vi "Report Error to Process.vi"(8 "Error":errorcluster, 11 "This VI":refnum<vi>) -> ()   [LabVIEW 2014, in "Waveform-Processing-Custom-Device Engine.lvlib" / "Error Handling API.lvlib"]
uses:
  Error Handling API.lvlib
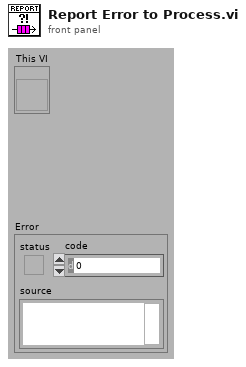
[diagram p1: front panel]
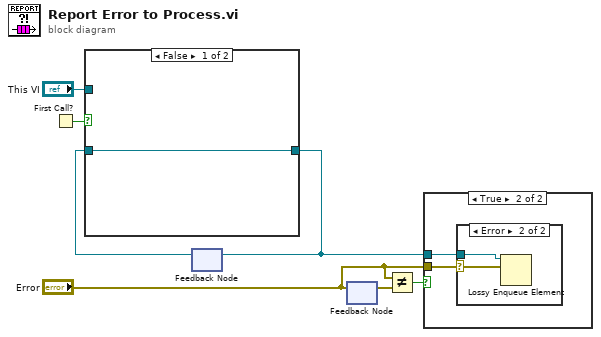
[diagram p0: block diagram]
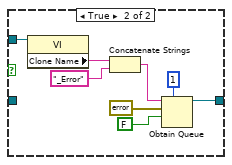
[diagram p4: hidden frame]
diagram:
  n1 = First Call?() -> (First Call?: T/F=w7:bool)
  n2 = feedback #1() -> (w5:refnum<queue>)  [unwired: 1 in]
  n3 = case shown="False" w7 {
    tunnel: "This VI" -> [_ w16]
    tunnel: [w8 w9] -> w1
    tunnel: w5 -> [w8 _]
    frame False {
    }
    frame True {
      n4 = property class="VI"(reference=w16) -> ("Clone Name"=w15:string)  [unwired: 1 in, 2 out]
      n5 = Concatenate Strings(w15, "_Error" ("string")) -> (w13:string)
      n6 = Obtain Queue(max queue size (-1, unlimited)=1, name (unnamed)=w13, element data type=errorcluster {"status"=FALSE, "code"=0, "source"=""} ("error out"), create if not found? (T)=FALSE) -> (queue out=w9:refnum<queue>)  [unwired: 1 in, 2 out]
    }
  }
  n7 = feedback-in #1(w1) -> ()
  n8 = feedback #2() -> (w3:errorcluster)  [unwired: 1 in]
  n9 = feedback-in #2("Error") -> ()
  n10 = Not Equal?(x="Error", y=w3) -> (x != y?=w4:bool)
  n11 = case shown="True" w4 {
    tunnel: w1 -> [_ w18]
    tunnel: "Error" -> [_ w17]
    frame False {
    }
    frame True {
      n12 = case shown="Error" w17 {
        selector: w17 -> [_ w19]
        tunnel: w18 -> [_ w20]
        frame No Error {
        }
        frame Error {
          n13 = Lossy Enqueue Element(queue=w20, element=w19) -> ()  [unwired: 1 in, 4 out]
        }
      }
    }
  }
